vi "Increment.vi"(8 "error in (no error)":errorcluster, 10 "Step (1)":i32=1, 11 "LargeScrollbar in":refnum<class "LargeScrollbar.lvclass">) -> (0 "error out":errorcluster)   [LabVIEW 2015, in "LargeScrollbar.lvclass"]
doc: "<b> </b> <b> </b>\n©2016 Q Software Innovations, LLC (QSI)\nwritten by Quentin Alldredge\nproduced in LabVIEW 2015\n\nsupport@qsoftwareinnovations.com\nwww.qsoftwareinnovations.com\n\nAll rights reserved.\n\nRedistribution and use in source and binary forms, with or without modification, are permitted provided that the following conditions are met:\n\n * Redistributions of source code must retain the above copyright notice, this list of conditions and the following disclaimer.\n * Redistributions in binary form must reproduce the above copyright notice, this list of conditions and the following disclaimer in the documentation and/or other materials provided with the distribution.\n * Neither the name of Q Software Innovations, LLC. nor the names of its contributors may be used to endorse or promote products derived from this software without specific prior written permission.\n\nTHIS SOFTWARE IS PROVIDED BY THE COPYRIGHT HOLDERS AND CONTRIBUTORS \"AS IS\" AND ANY EXPRESS OR IMPLIED WARRANTIES, INCLUDING, BUT NOT LIMITED TO, THE IMPLIED WARRANTIES OF MERCHANTABILITY AND FITNESS FOR A PARTICULAR PURPOSE ARE DISCLAIMED. IN NO EVENT SHALL THE COPYRIGHT OWNER OR CONTRIBUTORS BE LIABLE FOR ANY DIRECT, INDIRECT, INCIDENTAL, SPECIAL, EXEMPLARY, OR CONSEQUENTIAL DAMAGES (INCLUDING, BUT NOT LIMITED TO, PROCUREMENT OF SUBSTITUTE GOODS OR SERVICES; LOSS OF USE, DATA, OR PROFITS; OR BUSINESS INTERRUPTION) HOWEVER CAUSED AND ON ANY THEORY OF LIABILITY, WHETHER IN CONTRACT, STRICT LIABILITY, OR TORT (INCLUDING NEGLIGENCE OR OTHERWISE) ARISING IN ANY WAY OUT OF THE USE OF THIS SOFTWARE, EVEN IF ADVISED OF THE POSSIBILITY OF SUCH DAMAGE."
uses:
  LargeScrollbar.lvclass
  Direction.ctl
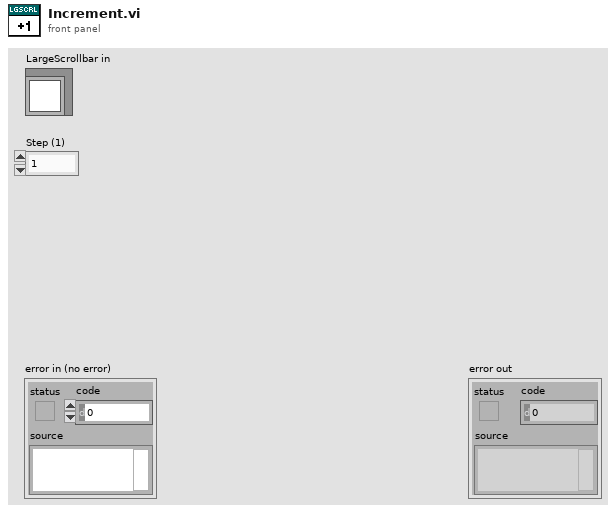
[diagram p1: front panel]
types:
  T1 = typedef "LargeScrollbar.lvclass/Direction.ctl" = enum16{"Decrement", "Increment"}
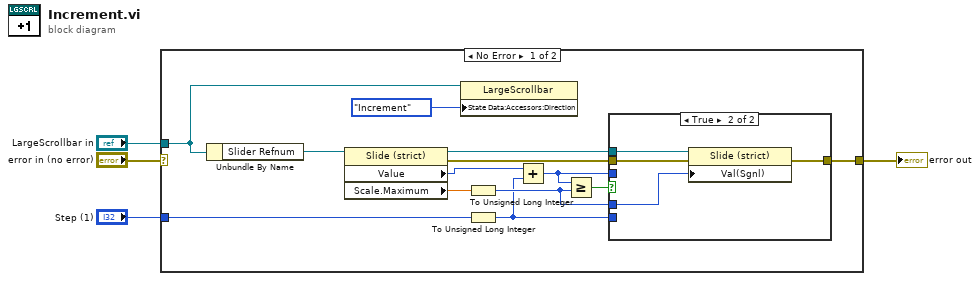
[diagram p0: block diagram]
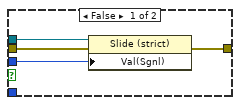
[diagram p2: hidden frame]
diagram:
  n1 = case shown="No Error" "error in (no error)" {
    selector: "error in (no error)" -> [_ w26]
    tunnel: [w14 w26] -> w3
    tunnel: "LargeScrollbar in" -> [w5 _]
    tunnel: "Step (1)" -> [w9 _]
    frame No Error {
      n2 = Unbundle By Name(w5) -> ("Slider Refnum"=w17:refnum<vi>)
      n3 = property class="Slide (strict)"(reference=w17) -> (reference out=w16:refnum<vi>, error out=w15:errorcluster, "Value"=w10:u32, "Scale.Maximum"=w13:dbl)  [unwired: 1 in]
      n4 = property class="LargeScrollbar"(reference=w5, "State Data:Accessors:Direction"=Direction."Increment" ("Direction")) -> ()  [unwired: 1 in, 2 out]
      n5 = To Unsigned Long Integer(number=w13) -> (unsigned 32bit integer=w8:u32)
      n6 = To Unsigned Long Integer(number=w9) -> (unsigned 32bit integer=w7:u32)
      n7 = Add(x=w10, y=w7) -> (x+y=w11:u32)
      n8 = Greater Or Equal?(x=w11, y=w8) -> (x >= y?=w12:bool)
      n9 = case shown="True" w12 {
        tunnel: w16 -> [w21 w25]
        tunnel: w15 -> [w20 w24]
        tunnel: [w19 w23] -> w14
        tunnel: w11 -> [w18 _]
        tunnel: w7 -> [_ _]
        tunnel: w8 -> [_ w22]
        frame False {
          n10 = property class="Slide (strict)"(reference=w21, error in=w20, "Val(Sgnl)"=w18) -> (error out=w19:errorcluster)  [unwired: 1 out]
        }
        frame True {
          n11 = property class="Slide (strict)"(reference=w25, error in=w24, "Val(Sgnl)"=w22) -> (error out=w23:errorcluster)  [unwired: 1 out]
        }
      }
    }
    frame Error {
    }
  }
  "error out" <- w3
